vi "Cleanup.vi"(8 "error in (no error)":errorcluster, 11 "Node in":refnum<class "abs_Type Leaf.lvclass">) -> (0 "error out":errorcluster, 3 "Node out":refnum<class "abs_Type Leaf.lvclass">)   [LabVIEW 2021, in "BT AbsType.lvlib" / "abs_Type Leaf.lvclass"]
uses:
  abs_Type Leaf.lvclass
  abs_Type Leaf.lvclass/abs_Type Leaf.ctl
  <vilib>/TSA/Abstract Data Classes/Abs_Types/Type/Abs_Type.lvclass
  Source/Support/Nodes/Leaves/Leaf/bt_Leaf.lvclass
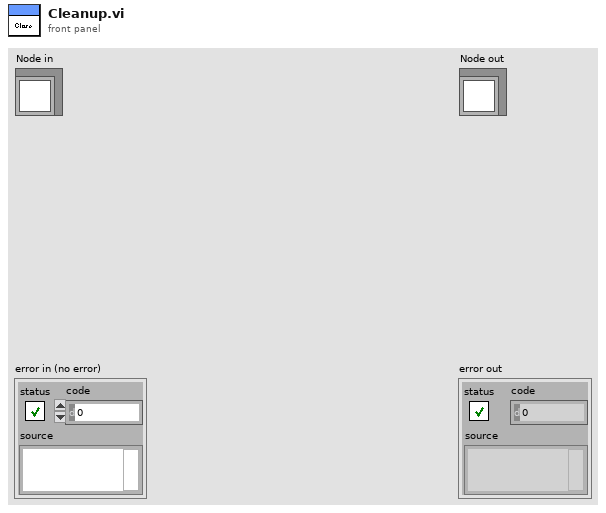
[diagram p1: front panel]
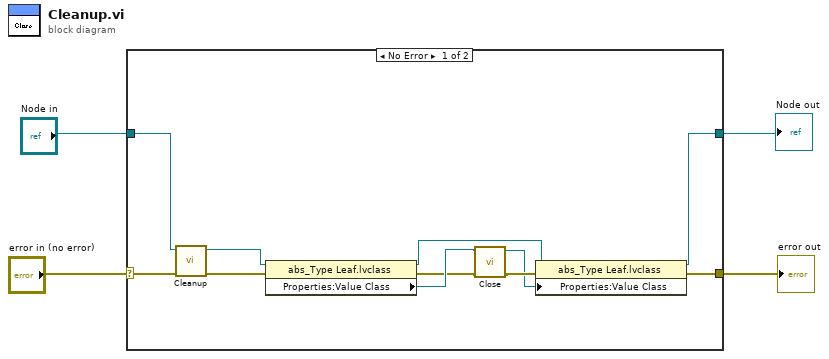
[diagram p0: block diagram]
diagram:
  n1 = case shown="No Error" "error in (no error)" {
    selector: "error in (no error)" -> [w15 w16]
    tunnel: "Node in" -> [w14 w17]
    tunnel: [w10 w16] -> w4
    tunnel: [w9 w17] -> w2
    frame No Error {
      n2 = call-parent "Cleanup.vi"("error in (no error)"=w15, "Node in"=w14) -> ("error out"=w13:errorcluster, "Node out"=w12:refnum<class "abs_Type Leaf.lvclass">)  [unwired: 8 in]
      n3 = property class="abs_Type Leaf.lvclass"(reference=w12, error in=w13) -> (reference out=w11:refnum<class "abs_Type Leaf.lvclass">, error out=w7:errorcluster, "Properties:Value Class"=w8:refnum<class "Abs_Type.lvclass">)
      n4 = call-dynamic "Close.vi"("error in (no error)"=w7, "Data in"=w8) -> ("error out"=w6:errorcluster, "Data out"=w5:refnum<class "Abs_Type.lvclass">)  [unwired: 8 in]
      n5 = property class="abs_Type Leaf.lvclass"(reference=w11, error in=w6, "Properties:Value Class"=w5) -> (reference out=w9:refnum<class "abs_Type Leaf.lvclass">, error out=w10:errorcluster)
    }
    frame Error {
    }
  }
  "error out" <- w4
  "Node out" <- w2
